vi "扫描测试数据保存.vi"(8 "错误输入（无错误）":errorcluster, 10 "扫描数据":dbl[][](array[numeric]), 11 "start path":path=path "D:/Data") -> (0 "错误输出":errorcluster)   [LabVIEW 2020]
uses:
  <vilib>/Utility/file.llb/Write Delimited Spreadsheet (DBL).vi
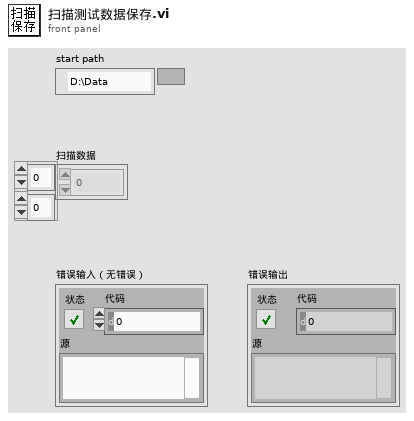
[diagram p1: front panel]
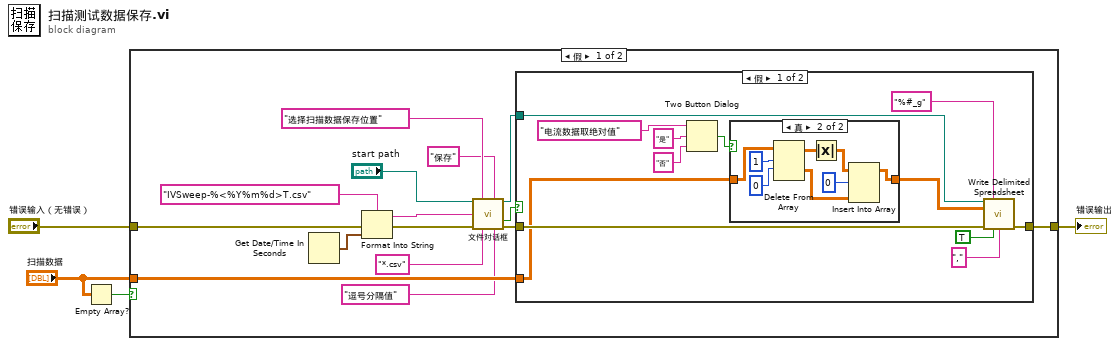
[diagram p0: block diagram]
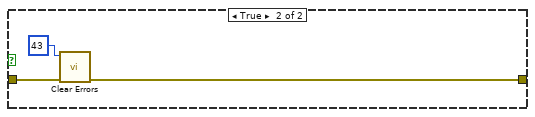
[diagram p3: hidden frame]
diagram:
  n1 = Empty Array?(array="扫描数据") -> (empty?=w1:bool)
  n2 = case shown="假" w1 {
    tunnel: "扫描数据" -> [w18 _]
    tunnel: [w16 w44] -> w4
    tunnel: "错误输入（无错误）" -> [w13 w44]
    frame False {
      n3 = Get Date/Time In Seconds() -> (seconds since 1Jan1904=w7:timestamp)
      n4 = Format Into String(format string="IVSweep-%<%Y%m%d>T.csv" ("格式字符串"), error in=w13, w7) -> (resulting string=w9:string, error out=w8:errorcluster)  [unwired: 1 in]
      n5 = call "文件对话框"("start path"="start path", "prompt"="选择扫描数据保存位置", "button label"="保存", "default name"=w9, "error in"=w8, "pattern (all files)"="*.csv", "pattern label"="逗号分隔值") -> ("selected path"=w17:path, "cancelled"=w19:bool, "error out"=w14:errorcluster)  [unwired: 5 in, 1 out]
      n6 = case shown="假" w19 {
        tunnel: w14 -> [w31 w43]
        tunnel: [w30 w42] -> w16
        tunnel: w17 -> [w29 _]
        tunnel: w18 -> [w22 _]
        frame False {
          n7 = Two Button Dialog(message="电流数据取绝对值" ("消息"), 1:"否" ("F按钮名称（“取消”）"), 2:"是" ("T按钮名称（“确定”）")) -> (T button?=w21:bool)
          n8 = case shown="真" w21 {
            tunnel: w22 -> [w32 w36]
            tunnel: [w32 w35] -> w20
            frame False {
            }
            frame True {
              n9 = Delete From Array(array=w36, length=1 ("长度"), index (row)=0 ("禁用的索引 (列)")) -> (deleted portion=w37:dbl[][], array with subset deleted=w39:dbl[][])  [unwired: 1 in]
              n10 = Absolute Value(x=w39) -> (abs(x)=w38:dbl[][])
              n11 = Insert Into Array(array=w38, index (row)=0 ("禁用的索引 (列)"), new element=w37) -> (w35:dbl[][])  [unwired: 1 in]
            }
          }
          n12 = call-poly <vilib>:"Write Delimited Spreadsheet.vi"("file path (dialog if empty)"=w29, "format (%.3f)"="%#_g", "2D data"=w20, "error in (no error)"=w31, "transpose? (no:F)"=TRUE, "delimiter (\\t)"="," ("delimiter (\\t)")) -> ("error out"=w30:errorcluster)  [unwired: 8 in, 1 out]
        }
        frame True {
          n13 = call <vilib>:"Clear Errors.vi"("error in (no error)"=w43, "specific error code to clear (0: all)"=43) -> ("error out"=w42:errorcluster)  [unwired: 4 in, 1 out]
        }
      }
    }
    frame True {
    }
  }
  "错误输出" <- w4
